vi "Write Clicked.vi"(8 "error in (no error)":errorcluster, 10 "Clicked":bool, 11 "Rectangle3D in":refnum<class "Rectangle3D.lvclass">) -> (0 "error out":errorcluster, 3 "Rectangle3D out":refnum<class "Rectangle3D.lvclass">)   [LabVIEW 2016, in "Rectangle3D.lvclass"]
uses:
  Rectangle3D.lvclass
  Rectangle3D.lvclass/Rectangle3D.ctl
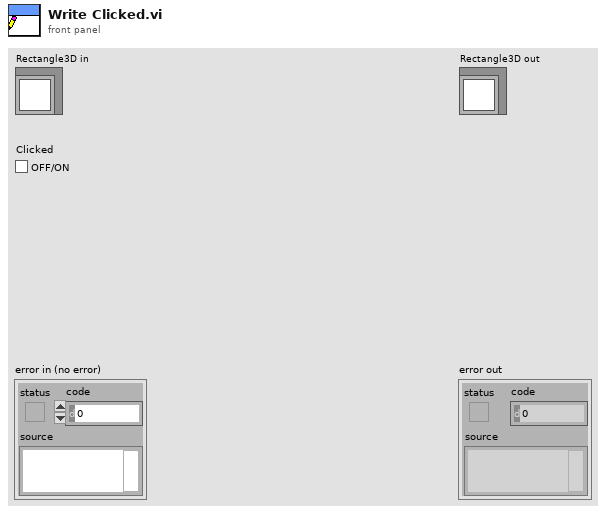
[diagram p1: front panel]
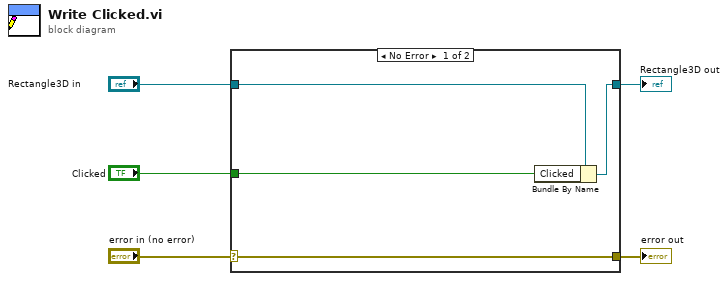
[diagram p0: block diagram]
diagram:
  n1 = case shown="No Error" "error in (no error)" {
    selector: "error in (no error)" -> [w9 w10]
    tunnel: [w9 w10] -> w4
    tunnel: [w7 w11] -> w2
    tunnel: "Rectangle3D in" -> [w8 w11]
    tunnel: "Clicked" -> [w6 _]
    frame No Error {
      n2 = Bundle By Name(cluster=w8, "Clicked"=w6) -> (w7:refnum<class "Rectangle3D.lvclass">)
    }
    frame Error {
    }
  }
  "error out" <- w4
  "Rectangle3D out" <- w2
